vi "电动工具串口配置.vi"() -> (5 "VISA resource name out":refnum<visa-resource-name> caption="VISA资源名称输出")   [LabVIEW 2013]
uses:
  <vilib>/Instr/_visa.llb/VISA Configure Serial Port (Instr).vi
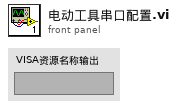
[diagram p1: front panel]
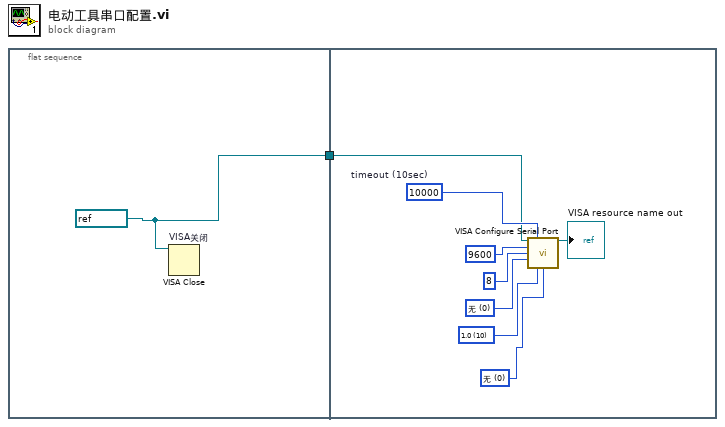
[diagram p0: block diagram]
diagram:
  n1 = flat-sequence {
    tunnel: [w2] -> w1
    tunnel: w1 -> [w5]
    frame #0 {
      w2 = refnum<visa-resource-name> "COM9" ("VISA resource name")
      n2 = VISA Close "VISA关闭"(VISA resource name=w2) -> ()  [unwired: 1 in, 1 out]
    }
    frame #1 {
      w3 = u16 0 items=["无", "XON/XOFF", "RTS/CTS", "XON/XOFF & RTS/CTS", "DTR/DSR", "XON/XOFF & DTR/DSR"] ("flow control (0:none)")
      w9 = u16 10 items=["1.0"=10, "1.5"=15, "2.0"=20] ("stop bits")
      w7 = u16 0 items=["无", "奇", "偶", "标记", "空格"] ("parity")
      w8 = u32 10000  # timeout (10sec)
      n3 = call-poly "VISA Configure Serial Port"("VISA resource name"=w5, "timeout (10sec)"=w8, "baud rate (9600)"=u32 9600 ("baud rate"), "data bits (8)"=u16 8 ("data bits"), "parity (0:none)"=w7, "stop bits (10: 1 bit)"=w9, "flow control (0:none)"=w3) -> ("VISA resource name out"=→"VISA resource name out":refnum<visa-resource-name>)  [unwired: 2 in, 6 out]
    }
  }
